vi "DAQ.GetPublicEvents.vi"(8 "error in (no error)":errorcluster, 11 "Instrument.DAQ":refnum<class "Instrument.DAQ.lvclass">) -> (0 "error out":errorcluster, 2 "DAQ Public Events":T1, 3 "Instrument.DAQ out":refnum<class "Instrument.DAQ.lvclass">)   [LabVIEW 2019, in "Instrument.Lockin.lvlib" / "Instrument.DAQ.lvclass"]
doc: "---------------------------------------------------------------\nJKI State Machine Objects™\nhttp://jki.net/state-machine-objects/\nCopyright (C) 2005-2015, JKI <info@jki.net>\nALL RIGHTS RESERVEDJKI State Machine Objects (SMO) 1.0.0.4\nJKI - JKI\nCopyright (c) 2015, JKI"
uses:
  Instrument.DAQ.lvclass
  Typedefs/PublicEvents--Cluster.ctl
  Typedefs/PublicEvents--DAQ.getAIChannels.ctl
  Typedefs/AI.Channel--Cluster--Array.ctl
  Typedefs/AI.Channel--Cluster.ctl
  Typedefs/PublicEvents--DAQ.getAOChannels.ctl
  Typedefs/AO.Channel--Cluster--Array.ctl
  Typedefs/AO.Channel--Cluster.ctl
  Typedefs/AO.Channel.Function--Enum.ctl
  Typedefs/PublicEvents--DAQ.getREFChannels.ctl
  Typedefs/REF.Channel--Cluster--Array.ctl
  Typedefs/REF.Channel--Cluster.ctl
  Typedefs/PublicEvents--DAQ.getWaveforms.ctl
  Typedefs/PublicEvents--DAQ.getResults.ctl
  Typedefs/Results--Cluster.ctl
  Typedefs/PublicEvents--DAQ.getSweepWaveforms.ctl
  Typedefs/PublicEvents--DAQ.getCalibration.ctl
  Typedefs/DAQ.Calibration--Cluster--Array.ctl
  Typedefs/DAQ.Calibration--Cluster.ctl
  Typedefs/PublicEvents--DAQ.getDAQState.ctl
  Typedefs/Status--enum.ctl
  Typedefs/PublicEvents--DAQ.getDAQconfig.ctl
  Typedefs/DAQ.Configuration--Cluster--Array.ctl
  Typedefs/DAQ.Configuration--Cluster.ctl
  Typedefs/DAQ.Config.AO.Range--enum.ctl
  Typedefs/DAQ.TerminalConfiguration--ring.ctl
  Typedefs/DAQ.Config.AI.Range--enum.ctl
  Typedefs/DAQ.Config.AI.Coupling--enum.ctl
  Typedefs/PublicEvents--DAQ.getInputGain.ctl
  Typedefs/Channel.Gain--Cluster--Array.ctl
  Typedefs/Channel.Gain--Cluster.ctl
  Typedefs/PublicEvents--DAQ.getOutputGain.ctl
  Typedefs/PublicEvents--DAQ.getInputOffset.ctl
  Typedefs/PublicEvents--DAQ.getSampling.ctl
  Typedefs/DAQ.Sampling--Cluster.ctl
  Typedefs/DAQ.Sampling.Sampling--Cluster.ctl
  Typedefs/PublicEvents--DAQ.getSweepChannels.ctl
  Typedefs/Sweep.Configuration--Cluster.ctl
  Typedefs/Sweep.Channel--Cluster--Array.ctl
  Typedefs/Sweep.Channel--Cluster.ctl
  Typedefs/Sweep.Pattern--Enum.ctl
  Typedefs/PublicEvents--DAQ.getDeviceIDN.ctl
  Typedefs/DeviceInfo--Cluster.ctl
  Instrument.DAQ.lvclass/Instrument.DAQ.ctl
panel:
  # "For instructions on how to use the JKI State Machine Objects, examples and video tutorials, visit:\nhttp://jki.net/state-machine-objects/\n\nJKI State Machine Objects™\nhttp://jki.net/state-machine-objects/\nCopyright (C) 2005-2015, JKI <info@jki.net>\nALL RIGHTS RESERVED"
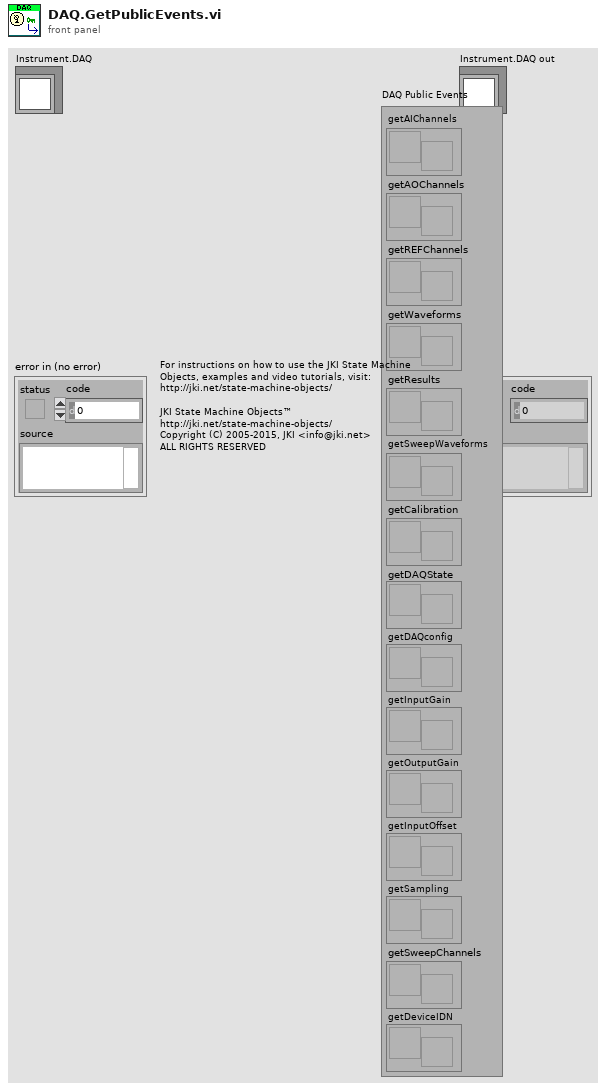
[diagram p1: front panel]
types:
  T1 = typedef "Instrument.Lockin.lvlib/Instrument.DAQ.lvclass/PublicEvents--Cluster.ctl" = cluster{"getAIChannels":refnum<user-event>, "getAOChannels":refnum<user-event>, "getREFChannels":refnum<user-event>, "getWaveforms":refnum<user-event>, "getResults":refnum<user-event>, "getSweepWaveforms":refnum<user-event>, "getCalibration":refnum<user-event>, "getDAQState":refnum<user-event>, "getDAQconfig":refnum<user-event>, "getInputGain":refnum<user-event>, "getOutputGain":refnum<user-event>, "getInputOffset":refnum<user-event>, "getSampling":refnum<user-event>, "getSweepChannels":refnum<user-event>, "getDeviceIDN":refnum<user-event>}
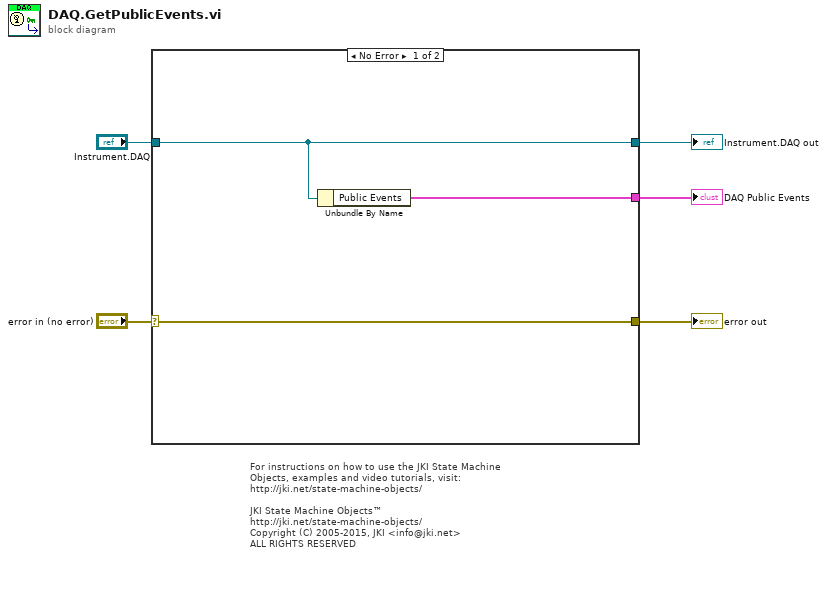
[diagram p0: block diagram]
diagram:
  # "For instructions on how to use the JKI State Machine Objects, examples and video tutorials, visit:\nhttp://jki.net/state-machine-objects/\n\nJKI State Machine Objects™\nhttp://jki.net/state-machine-objects/\nCopyright (C) 2005-2015, JKI <info@jki.net>\nALL RIGHTS RESERVED"
  n1 = case shown="No Error" "error in (no error)" {
    selector: "error in (no error)" -> [w7 w9]
    tunnel: "Instrument.DAQ" -> [w6 w10]
    tunnel: [w7 w9] -> w4
    tunnel: [w6 w10] -> w3
    tunnel: [w8 _] -> w1
    frame No Error {
      n2 = Unbundle By Name(w6) -> ("Public Events"=w8:T1)
    }
    frame Error {
    }
  }
  "error out" <- w4
  "Instrument.DAQ out" <- w3
  "DAQ Public Events" <- w1
